vi "Complete Request.vi"(7 "Processing In":refnum<class "Processing.lvclass">, 11 "Caching Complete in":refnum<class "Caching Complete.lvclass">) -> (0 "error out":errorcluster, 5 "Processing":refnum<class "Processing.lvclass">)   [LabVIEW 2020, in "HTTP Server.lvlib" / "Caching Complete.lvclass"]
uses:
  Caching Complete.lvclass
  Processing/Processing.lvclass
  Caching Complete.lvclass/Caching Complete.ctl
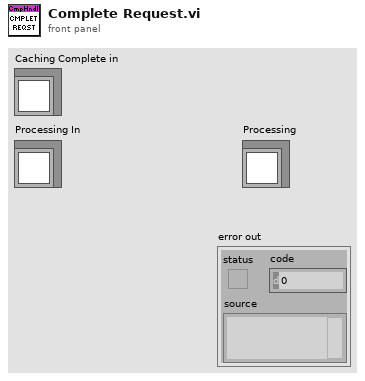
[diagram p1: front panel]
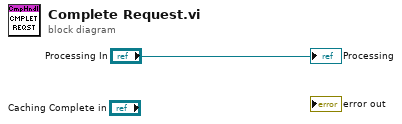
[diagram p0: block diagram]
diagram:
  "Processing" <- "Processing In"
